vi "DrawSpaceship.vi"(8 "error in":errorcluster, 10 "InitCluster_IN":T1) -> (0 "error out":errorcluster, 2 "InitCluster_OUT":T1, 3 "SpaceshipPosition":T7)   [LabVIEW 2019]
uses:
  InitCluster.ctl
  CharacterCluster.ctl
  <vilib>/picture/picture.llb/imagedata.ctl
  ShotInitCluster.ctl
  <vilib>/Utility/miscctls.llb/LVPositionTypeDef.ctl
  <vilib>/Utility/miscctls.llb/LVBoundsTypeDef.ctl
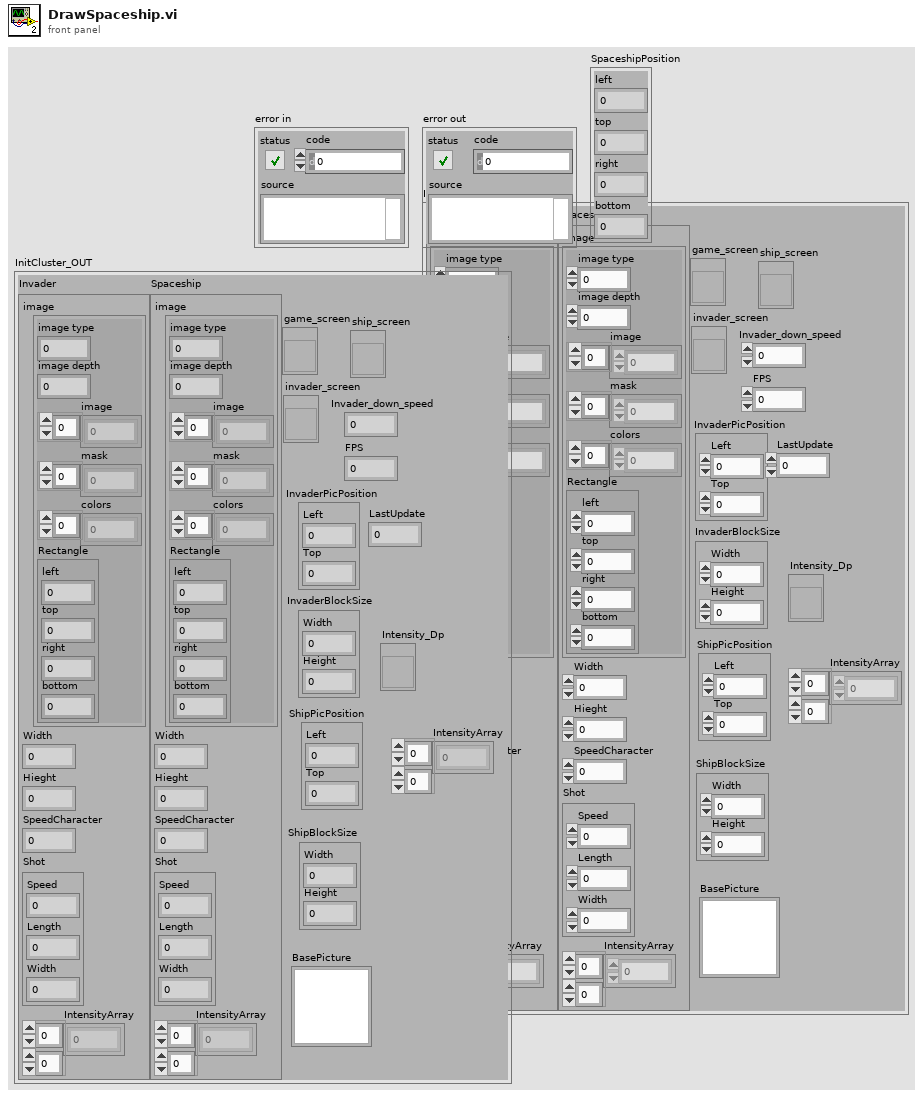
[diagram p1: front panel]
types:
  T1 = typedef "InitCluster.ctl" = cluster{"Invader":T2, "Spaceship":T2, "game_screen":refnum<vi>, "BasePicture":picture, "invader_screen":refnum<vi>, "InvaderPicPosition":T5, "Invader_down_speed":i16, "FPS":u16, "InvaderBlockSize":T6, "ship_screen":refnum<vi>, "ShipBlockSize":T6, "ShipPicPosition":T5, "LastUpdate":u32, "Intensity_Dp":refnum<vi>, "IntensityArray":u8[][]}
  T2 = typedef "CharacterCluster.ctl" = cluster{"image":T3, "Width":u32, "Hieght":u32, "SpeedCharacter":u32, "Shot":T4, "IntensityArray":u8[][]}
  T3 = typedef "imagedata.ctl" = cluster{"image type":i32, "image depth":i32, "image":u8[], "mask":u8[], "colors":u32[], "Rectangle":cluster{"left":i16, "top":i16, "right":i16, "bottom":i16}}
  T4 = typedef "ShotInitCluster.ctl" = cluster{"Speed":u32, "Length":u32, "Width":u32}
  T5 = typedef "LVPositionTypeDef.ctl" = cluster{"Left":i32, "Top":i32}
  T6 = typedef "LVBoundsTypeDef.ctl" = cluster{"Width":u32, "Height":u32}
  T7 = cluster{"left":i16, "top":i16, "right":i16, "bottom":i16}
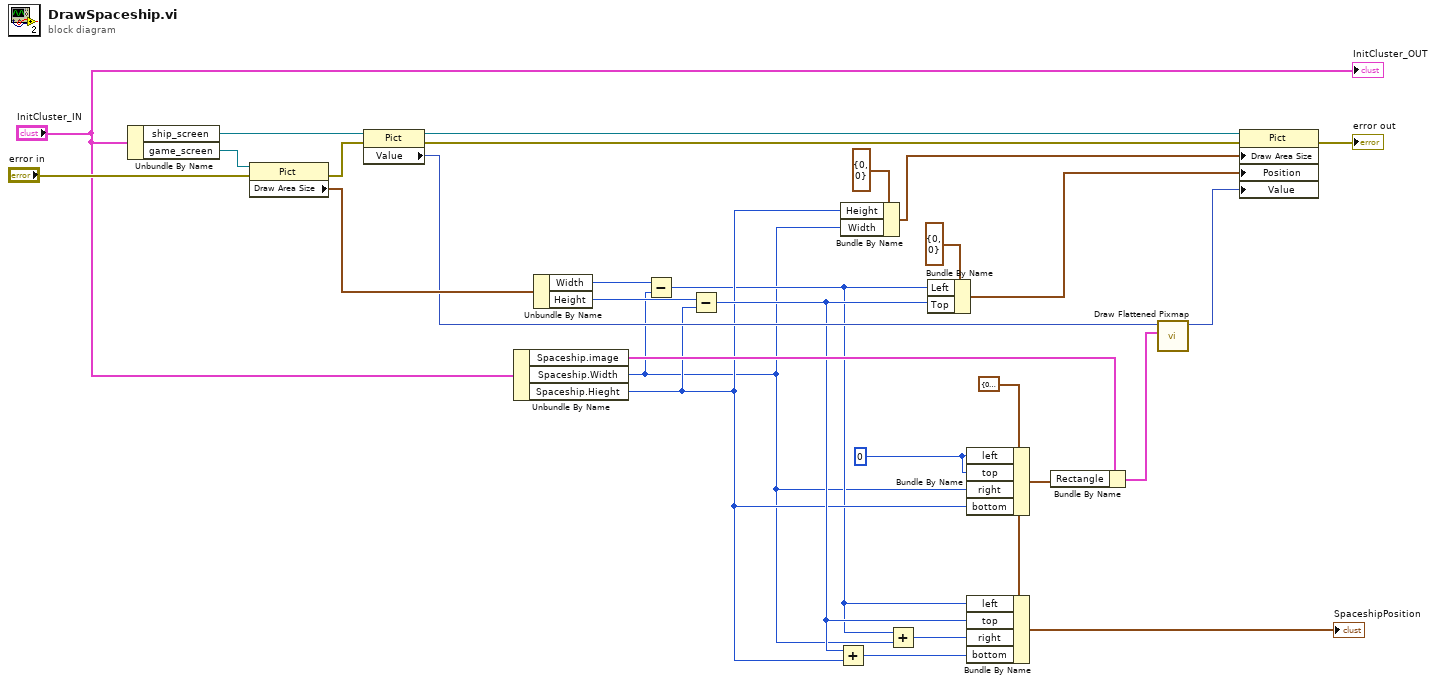
[diagram p0: block diagram]
diagram:
  w9 = i16 0 ("left")
  w8 = T7 {"left"=0, "top"=0, "right"=0, "bottom"=0} ("Rectangle")
  n1 = Unbundle By Name("InitCluster_IN") -> ("ship_screen"=w16:refnum<vi>, "game_screen"=w29:refnum<vi>)
  n2 = property class="Pict"(reference=w29, error in="error in") -> (error out=w14:errorcluster, "Draw Area Size"=w24:T6)  [unwired: 1 out]
  n3 = property class="Pict"(reference=w16, error in=w14) -> (reference out=w15:refnum<vi>, error out=w13:errorcluster, "Value"=w12:picture)
  n4 = Unbundle By Name("InitCluster_IN") -> ("Spaceship.image"=w26:T3, "Spaceship.Width"=w2:u32, "Spaceship.Hieght"=w6:u32)
  n5 = Unbundle By Name(w24) -> ("Width"=w11:u32, "Height"=w10:u32)
  n6 = Subtract(x=w11, y=w2) -> (x-y=w5:u32)
  n7 = Subtract(x=w10, y=w6) -> (x-y=w7:u32)
  n8 = Add(x=w7, y=w6) -> (x+y=w4:u32)
  n9 = Bundle By Name(cluster=T6 {"Width"=0, "Height"=0} ("Draw Area Size"), "Height"=w6, "Width"=w2) -> (w20:T6)
  n10 = Add(x=w5, y=w2) -> (x+y=w3:u32)
  n11 = Bundle By Name(cluster=T5 {"Left"=0, "Top"=0} ("Position"), "Left"=w5, "Top"=w7) -> (w17:T5)
  n12 = Bundle By Name(cluster=w8, "left"=w9, "top"=w9, "right"=w2, "bottom"=w6) -> (w23:T7)
  n13 = Bundle By Name(cluster=w8, "left"=w5, "top"=w7, "right"=w3, "bottom"=w4) -> (→"SpaceshipPosition":T7)
  n14 = Bundle By Name(cluster=w26, "Rectangle"=w23) -> (w25:T3)
  n15 = call <vilib>:"Draw Flattened Pixmap.vi"("image data"=w25, "picture"=w12) -> ("new picture"=w19:picture)  [unwired: 7 in]
  n16 = property class="Pict"(reference=w15, error in=w13, "Draw Area Size"=w20, "Position"=w17, "Value"=w19) -> (error out=→"error out":errorcluster)  [unwired: 1 out]
  "InitCluster_OUT" <- "InitCluster_IN"
